vi "X_AxisMotorControlSetupAndHome.vi"(11 "Automation Refnum in":refnum<k7>(container)) -> (2 "X Translation Serial Number":i32=40849496, 3 "Automation Refnum out":refnum<k7>)   [LabVIEW 2020]
panel:
  out "error out 2":errorcluster
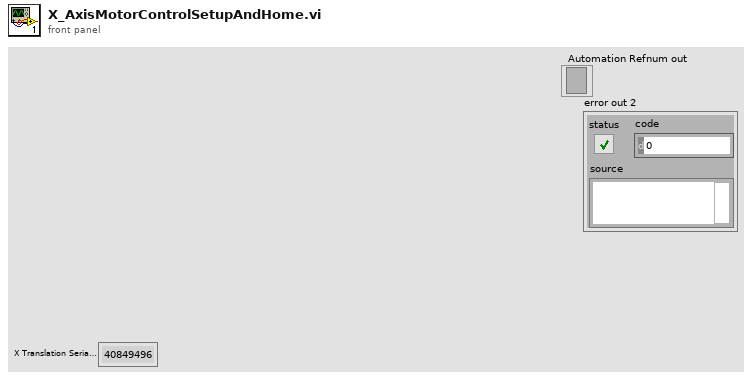
[diagram p1: front panel]
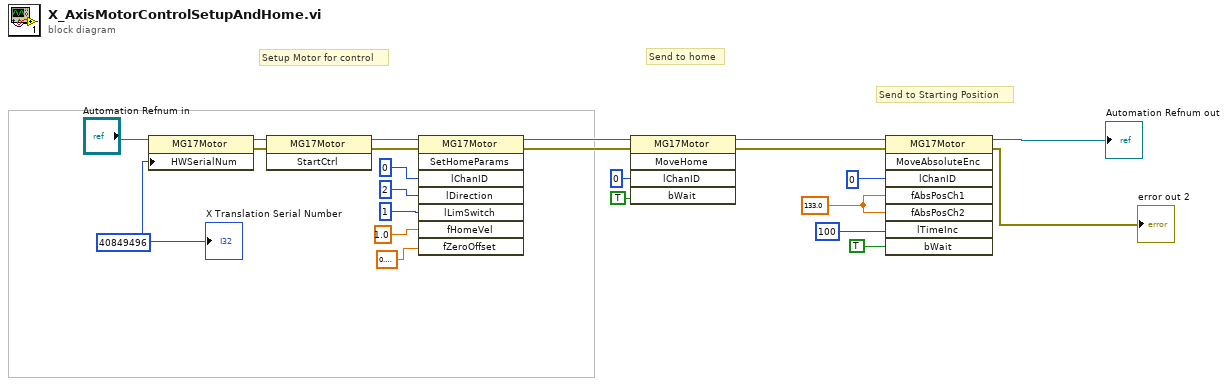
[diagram p0: block diagram]
diagram:
  w1 = sgl 133.0 ("fAbsPosCh1")
  w23 = 40849496 ("Serial Number")
  # "Send to Starting Position"
  # "Setup Motor for control"
  # "Send to home"
  n1 = property on="Property Node" class="MG17Motor"(reference="Automation Refnum in", "HWSerialNum"=w23) -> (reference out=w15:refnum<k7>, error out=w9:errorcluster)  [unwired: 1 in]
  n2 = invoke class="MG17Motor" method="StartCtrl"(reference=w15, error in=w9) -> (reference out=w13:refnum<k7>, error out=w10:errorcluster)  [unwired: 1 in, 1 out]
  n3 = invoke class="MG17Motor" method="SetHomeParams"(reference=w13, error in=w10, "lChanID"=0, "lDirection"=2, "lLimSwitch"=1, "fHomeVel"=sgl 1.0, "fZeroOffset"=sgl 0.1) -> (reference out=w12:refnum<k7>, error out=w11:errorcluster)  [unwired: 1 in, 6 out]
  n4 = invoke class="MG17Motor" method="MoveHome"(reference=w12, error in=w11, "lChanID"=0, "bWait"=TRUE) -> (reference out=w5:refnum<k7>, error out=w4:errorcluster)  [unwired: 1 in, 3 out]
  n5 = invoke class="MG17Motor" method="MoveAbsoluteEnc"(reference=w5, error in=w4, "lChanID"=0, "fAbsPosCh1"=w1, "fAbsPosCh2"=w1, "lTimeInc"=100, "bWait"=TRUE) -> (reference out=→"Automation Refnum out":refnum<k7>, error out=→"error out 2":errorcluster)  [unwired: 1 in, 6 out]
  "X Translation Serial Number" <- w23
